vi "MT Align To Ideal Symbols (FSK).vi"(0 "input phase waveform":cluster{"t0":dbl, "dt":dbl, "Y":cdb[]}={"t0"=0.0, "dt"=1.0, "Y"=[]} {"Y" format="%.3f"; "dt" format="%^.2e"; "t0" format="%.4f"}, 5 "matched filter coefficients":dbl[](array[numeric]) format="%^.2e", 7 "samples per symbol (16)":i32=16, 11 "error in (no error)":errorcluster, 13 "reset? (T)":bool=TRUE) -> (4 "output phase waveform":cluster{"t0":dbl, "dt":dbl, "Y":dbl[]} {"Y" min=0.0 max=127.0 format="%.3f"; "dt" format="%^.2e"; "t0" format="%.4f"}, 8 "waveform alignment offset (samples)":dbl, 15 "error out":errorcluster)   [LabVIEW 2020, in "niDMT.lvlib"]
doc: "This polymorphic instance aligns the first sample of the <B>input phase waveform</B> to the ideal symbol timing instant for an FSK modulation scheme."
uses:
  <vilib>/addons/Modulation/niDMT.lvlib
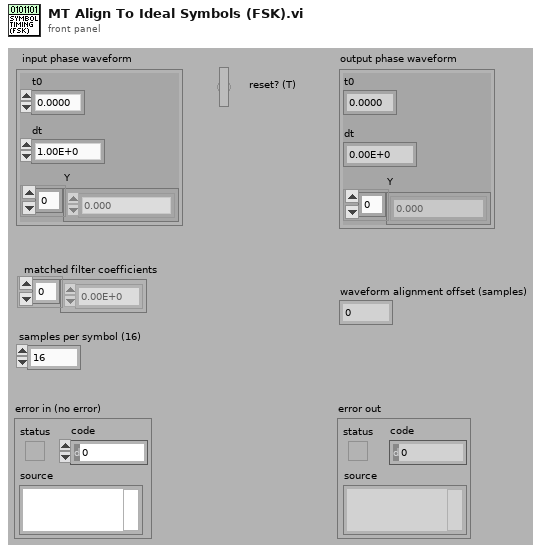
[diagram p1: front panel]
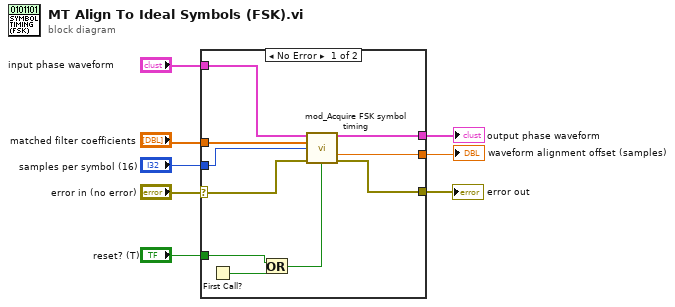
[diagram p0: block diagram]
diagram:
  n1 = case shown="No Error" "error in (no error)" {
    selector: "error in (no error)" -> [w9 w19]
    tunnel: "input phase waveform" -> [w18 _]
    tunnel: "matched filter coefficients" -> [w14 _]
    tunnel: "samples per symbol (16)" -> [w11 _]
    tunnel: "reset? (T)" -> [w17 _]
    tunnel: [w10 w19] -> w3
    tunnel: [w15 _] -> w2
    tunnel: [w13 _] -> w1
    frame No Error {
      n2 = First Call?() -> (First Call?: T/F=w16:bool)
      n3 = Or(x=w17, y=w16) -> (x .or. y?=w12:bool)
      n4 = call <vilib>:"mod_Acquire FSK symbol timing.vi"("input phase waveform"=w18, "matched filter coefficients"=w14, "samples per symbol (16)"=w11, "error in (no error)"=w9, "reset? (T)"=w12) -> ("output phase waveform"=w13:cluster{"t0":dbl, "dt":dbl, "Y":dbl[]}, "waveform alignment offset"=w15:dbl, "error out"=w10:errorcluster)  [unwired: 2 in, 6 out]
    }
    frame Error {
    }
  }
  "error out" <- w3
  "output phase waveform" <- w1
  "waveform alignment offset (samples)" <- w2
